vi "Create New EXE Extensions.vi"(7 "TargetItem Refnum":refnum<vi>, 8 "error in (no error)":errorcluster, 9 "Build specification name":string, 11 "Project Refnum":refnum<vi>) -> (0 "error out":errorcluster, 3 "NI_AB_API_Build out":refnum<class "NI_AB_API_EXE_Extensions.lvclass">)   [LabVIEW 2021, in "NI_AB_API_EXE_Extensions.lvclass"]
uses:
  NI_AB_API_EXE_Extensions.lvclass
  <vilib>/AppBuilder/AB_API/Build/NI_AB_API_Build.lvclass
  <vilib>/AppBuilder/AB_Classes/EXE/AB_EXE.lvclass
  <vilib>/AppBuilder/AB_API/common/AB_API Build Object Type.ctl
  C:/Program Files/National Instruments/LabVIEW 2021/vi.lib/AppBuilder/AB_Classes/Build/AB_Build.lvclass
  C:/Program Files/National Instruments/LabVIEW 2021/vi.lib/AppBuilder/AB_API/Build/NI_AB_API_Build.lvclass
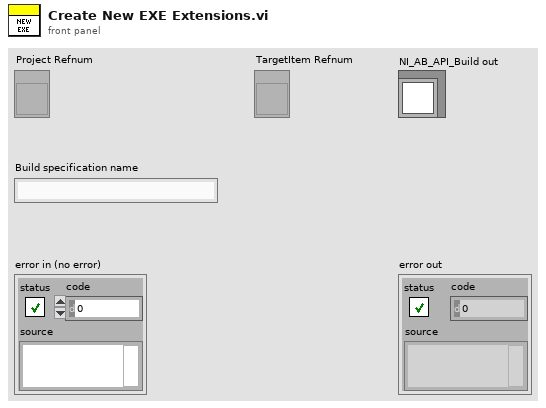
[diagram p1: front panel]
types:
  T1 = typedef "AB_API Build Object Type.ctl" = enum16{"Source Distribution", "DLL", "EXE", "Installer", "Zip File", "RESTful WS", "RTEXE", "Packed Library", "C Generation ", ".NET Interop Assembly"}
  T2 = typedef "ItemRef.ctl" = u64
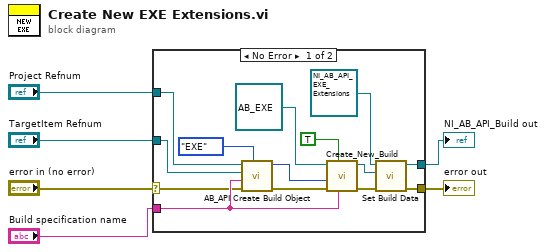
[diagram p0: block diagram]
diagram:
  n1 = case shown="No Error" "error in (no error)" {
    selector: "error in (no error)" -> [w9 w21]
    tunnel: [w13 w21] -> w5
    tunnel: [w11 _] -> w1
    tunnel: "Project Refnum" -> [w19 _]
    tunnel: "Build specification name" -> [w15 _]
    tunnel: "TargetItem Refnum" -> [w18 _]
    frame No Error {
      n2 = call <vilib>:"AB_API Create Build Object.vi"("Build object type"=AB_API_Build_Object_Type."EXE", "error in (no error)"=w9, "Build spec name"=w15, "TargetItem Refnum"=w18, "Project Refnum"=w19) -> ("error out"=w17:errorcluster, "Build object"=w16:T2)  [unwired: 5 out]
      n3 = call-dynamic "Create_New_Build.vi"("buildSpecName"=w15, "Programmatic? (false)"=TRUE, "error in (no error)"=w17, "buildObject"=w16, "AB_EXE in"=refnum<class "AB_EXE.lvclass"> refnum ("AB_EXE.lvclass")) -> ("error out"=w14:errorcluster, "AB_EXE out"=w12:refnum<class "AB_EXE.lvclass">)  [unwired: 1 in, 4 out]
      n4 = call <vilib>:"Set Build Data.vi"("error in (no error)"=w14, "AB_Build.lvclass"=w12, "NI_AB_API_Build in"=refnum<class "NI_AB_API_EXE_Extensions.lvclass"> refnum ("NI_AB_API_EXE_Extensions.lvclass")) -> ("error out"=w13:errorcluster, "NI_AB_API_Build out"=w11:refnum<class "NI_AB_API_EXE_Extensions.lvclass">)  [unwired: 7 in]
    }
    frame Error {
    }
  }
  "error out" <- w5
  "NI_AB_API_Build out" <- w1
